vi "CFG Insert Item.vi"(0 "Parameters":T1[](array[typedef]), 5 "Value":variant, 7 "Delimiter(s) (Empty: N/A)":string, 12 "Tag":string) -> (4 "Parameters":T1[](array[typedef]))   [LabVIEW 2017]
uses:
  Type Defs/CFG Key Cluster.ctl
  Type Defs/CFG Tag Type Enum.ctl
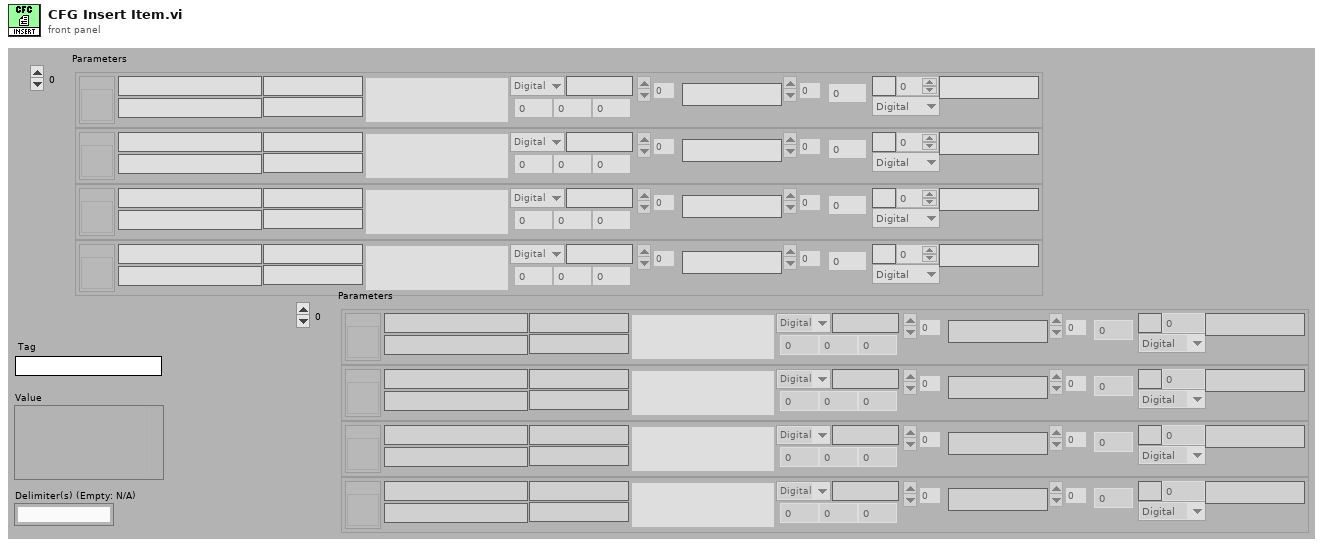
[diagram p1: front panel]
types:
  T1 = typedef "CFG Key Cluster.ctl" = cluster{"Strings []":string[], "Disabled Items []":i32[], "Value":variant, "Format String":string, "Tag":string, "Type":T2, "Section":string, " Ctl Ref":refnum<vi>, "Data Range":cluster{"Minimum":dbl, "Maximum":dbl, "Increment":dbl}, "Unit":string, "Special Instructions":string, "Delimiter(s)":string, "Dimensions":i32, "Element Type":T2, "Array Value String":string}
  T2 = typedef "CFG Tag Type Enum.ctl" = enum16{"Digital", "Slide", "Enum", "Boolean", "String", "Path", "Array", "VISAResourceName", "DAQmxName", "Cluster"}
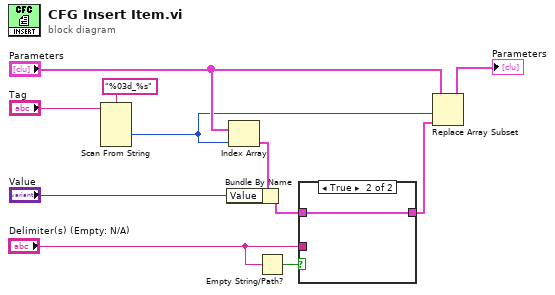
[diagram p0: block diagram]
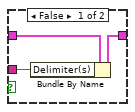
[diagram p2: hidden frame]
diagram:
  n1 = Scan From String(format string="%03d_%s", input string="Tag") -> (output 1=w6:i32)  [unwired: 2 in, 6 out]
  n2 = Index Array(array="Parameters", index=w6) -> (element=w9:T1)
  n3 = Bundle By Name(cluster=w9, "Value"="Value") -> (w4:T1)
  n4 = Empty String/Path?(string/path="Delimiter(s) (Empty: N/A)") -> (empty?=w1:bool)
  n5 = case shown="True" w1 {
    tunnel: w4 -> [w14 w15]
    tunnel: [w13 w15] -> w3
    tunnel: "Delimiter(s) (Empty: N/A)" -> [w12 _]
    frame False {
      n6 = Bundle By Name(cluster=w14, "Delimiter(s)"=w12) -> (w13:T1)
    }
    frame True {
    }
  }
  n7 = Replace Array Subset(array="Parameters", new element=w3, index=w6) -> (→"Parameters":T1[])
